vi "GT_GetAxisPrfVel.vi"(2 "Axis":T1=2 items=["Axis Control"=0, "Axis 1"=1, "Axis 2"=2, "Axis 3"=3, "Axis 4"=4, "Axis 5"=5, "Axis 6"=6, "Axis 7"=7, "Axis 8"=8, "Vector Space Control"=16, "Vector Space 1"=17, "Vector Space 2"=18, "Vector Space 3"=19, "Vector Space 4"=20], 3 "rtn_In":cluster{"rtn":i16, "Func":string}) -> (0 "pValue":dbl, 1 "rtn_Out":cluster{"rtn":i16, "Func":string})   [LabVIEW 2014]
uses:
  <vilib>/Motion/FlexMotion/CustomControls/CustomControls.llb/AxisOrVectorSpaceControl To Control.flx
  VC6/gts.dll
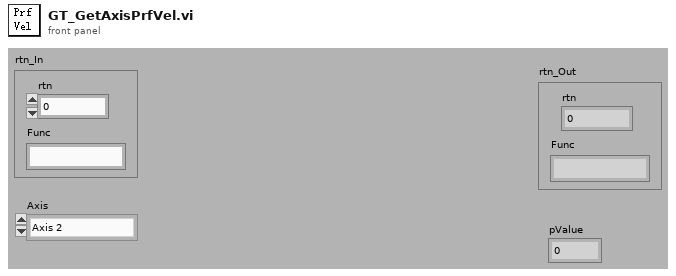
[diagram p1: front panel]
types:
  T1 = typedef "AxisOrVectorSpaceControl To Control.flx" = u16
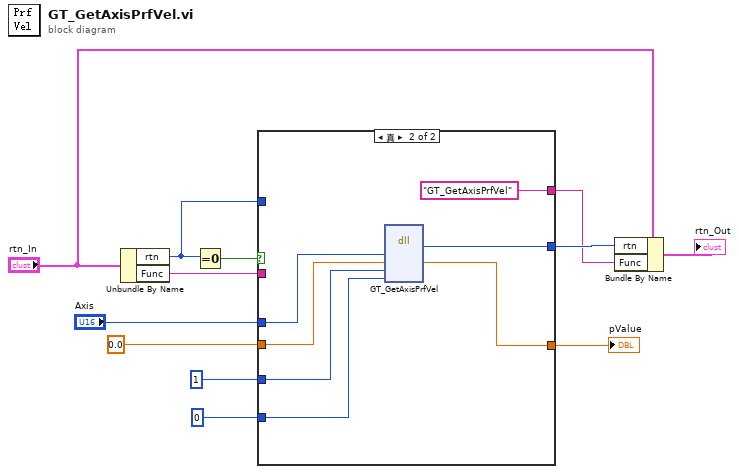
[diagram p0: block diagram]
diagram:
  n1 = Unbundle By Name("rtn_In") -> ("rtn"=w6:i16, "Func"=w11:string)
  n2 = Equal To 0?(x=w6) -> (x = 0?=w12:bool)
  n3 = case shown="真" w12 {
    tunnel: w11 -> [w14 _]
    tunnel: [w15 w22] -> w9
    tunnel: [w14 "GT_GetAxisPrfVel"] -> w7
    tunnel: w6 -> [w15 _]
    tunnel: "Axis" -> [_ w20]
    tunnel: 0.0 ("pValue") -> [w13 w19]
    tunnel: i16 1 ("count") -> [_ w18]
    tunnel: 0 ("pClock") -> [_ w17]
    tunnel: [w13 w16] -> w1
    frame False {
    }
    frame True {
      n4 = dll-call lib="PTH2Fabs DNewGTS AC-800LWin7版源程序-20170926gts85VC6gts.dll" fn="GT_GetAxisPrfVel"("axis"=w20, "pValue"=w19, "count"=w18, "pClock"=w17) -> ("rtn"=w22:i16, "pValue"=w16:dbl)  [unwired: 6 in, 2 out]
    }
  }
  "pValue" <- w1
  n5 = Bundle By Name(cluster="rtn_In", "rtn"=w9, "Func"=w7) -> (→"rtn_Out":cluster{"rtn":i16, "Func":string})
